vi "myRIO_BRig_RT__increment_u16.vi"() -> (2 "output_increment__u16":u16=5)   [LabVIEW 2014]
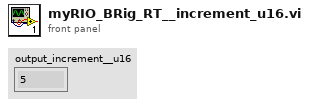
[diagram p1: front panel]
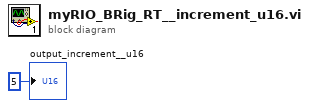
[diagram p0: block diagram]
diagram:
  "output_increment__u16" <- u16 5
